vi "Open.vi"(7 "I2C Channel":u8, 8 "Error In":errorcluster, 10 "I2C Slave Address (0)":u8, 11 "LINX Resource":T1) -> (0 "Error Out":errorcluster, 2 "Success?":bool, 3 "LINX Resource":T1)   [LabVIEW 2020, in "LMH-LINX.lvlib" / "MMA8451.lvlib"]
doc: "Open the I2C master and initialize the MMA8451 accelerometer with 14-bit resolution and +-2g mode.\n\nIf the LINX device has more than one I2C master the logical first I2C master is channel 0, the next is channel 1, etc.\n\nOrignal code contributed by SEbstein."
uses:
  MMA8451.lvlib
  Private/Type Defs/LINX Ref.ctl
  Private/Type Defs/Platform.ctl
  Private/Type Defs/Interface.ctl
  Private/Device/Type Defs/LINX Device Config.ctl
  Private/Device/Type Defs/TCP Config.ctl
  Private/Device/Type Defs/Channels.ctl
  Private/Type Defs/Peripherals/I2C/EOF.ctl
  Private/Local IO/LinxI2cWrite.vi
  Utilities/Check Channel.vi
  Private/Utilties/Generate Error.vi
  LMH-LINX.lvlib
  Private/Device/Device.lvlib
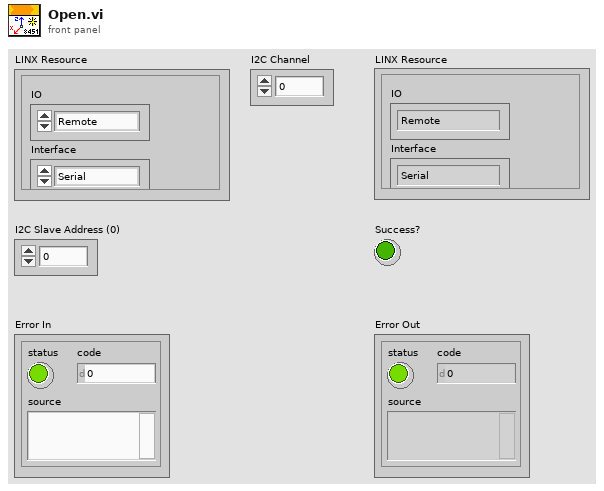
[diagram p1: front panel]
types:
  T1 = typedef "LMH-LINX.lvlib/LINX Ref.ctl" = cluster{"IO":T2, "Interface":T3, "LINX Device Config":T4}
  T2 = typedef "LMH-LINX.lvlib/Platform.ctl" = enum16{"Remote", "Local"}
  T3 = typedef "LMH-LINX.lvlib/Interface.ctl" = enum16{"Serial", "TCP"}
  T4 = typedef "Device.lvlib/LINX Device Config.ctl" = cluster{"Interface":T3, "COM Port":refnum<visa-resource-name>, "TCP Configuration":T5, "Device Family":u8, "Device ID":u8, "Device Name":string, "TCP Ref":refnum<k5>, "Channels":T6}
  T5 = typedef "Device.lvlib/TCP Config.ctl" = cluster{"IP Address":string, "Port":u16}
  T6 = typedef "LMH-LINX.lvlib/Channels.ctl" = cluster{"DI":u8[], "DO":u8[], "AI":u8[], "AO":u8[], "PWM":u8[], "QE":u8[], "UART":u8[], "I2C 2":u8[], "SPI":u8[], "CAN":u8[], "Servo":u8[], "AI Ref (V)":dbl, "AI Resolution (Bits)":u8, "AO Ref (V)":dbl, "AO Resolution (Bits)":u8}
  T7 = typedef "LMH-LINX.lvlib/EOF.ctl" = enum8{"Stop", "Restart", "Restart No Stop", "No Stop"}
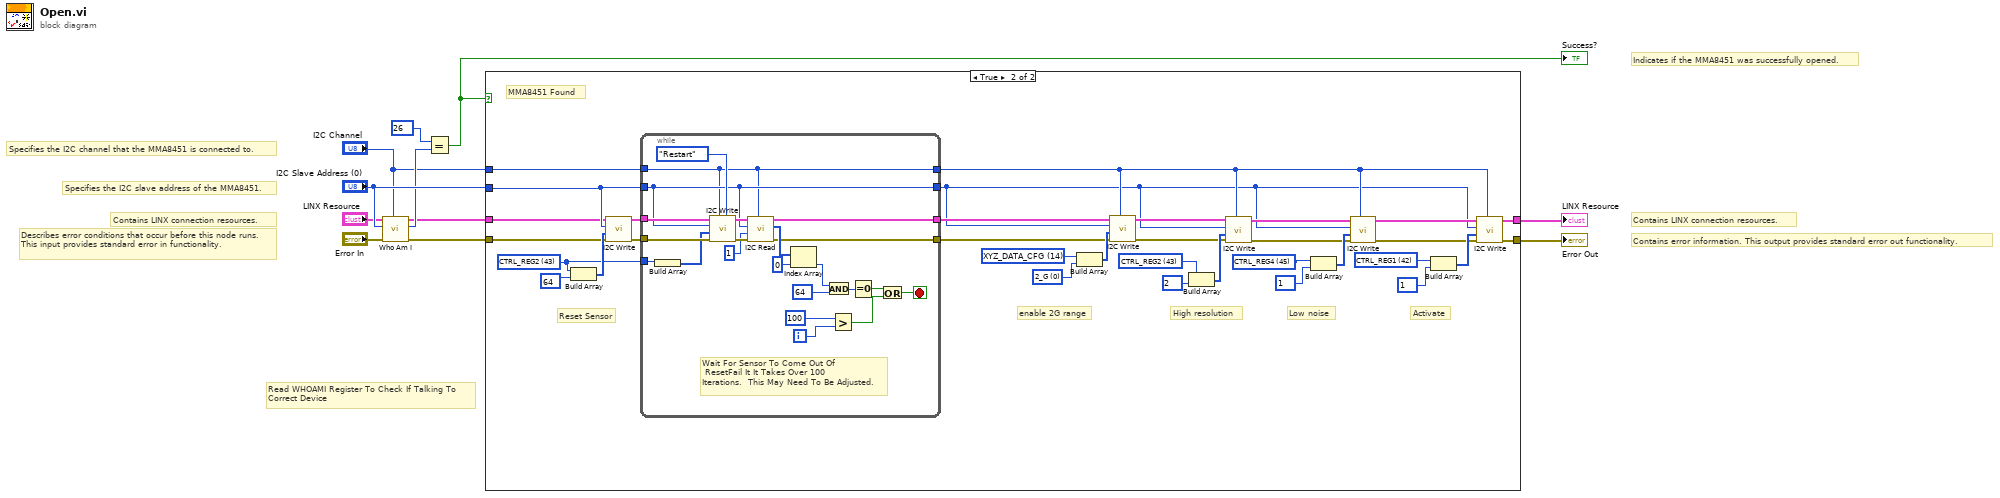
[diagram p0: block diagram]
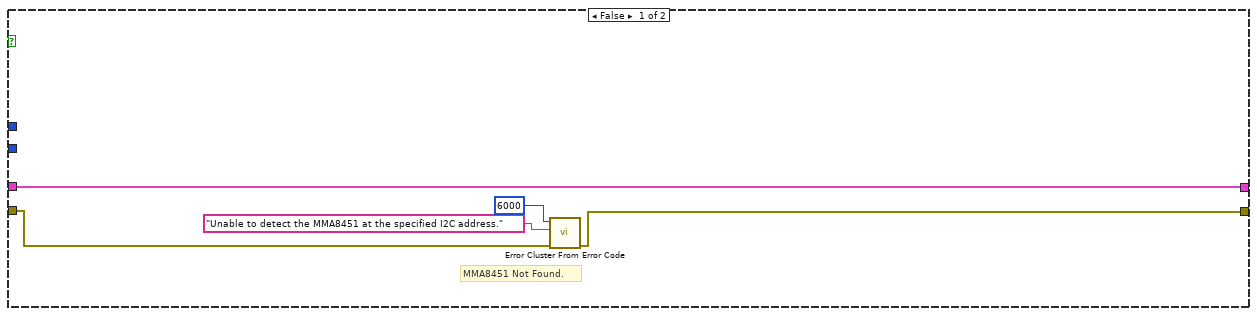
[diagram p2: hidden frame]
diagram:
  # "Indicates if the MMA8451 was successfully opened."
  # "Contains LINX connection resources."
  # "Contains error information. This output provides standard error out functionality."
  # "Specifies the I2C slave address of the MMA8451."
  # "Specifies the I2C channel that the MMA8451 is connected to."
  # "Contains LINX connection resources."
  # "Describes error conditions that occur before this node runs. This input provides standard error in functionality."
  # "Read WHOAMI Register To Check If Talking To \nCorrect Device"
  n1 = call "Who Am I.vi"("I2C Channel"="I2C Channel", "Error In"="Error In", "I2C Slave Address (0)"="I2C Slave Address (0)", "LINX Resource"="LINX Resource") -> ("Error Out"=w6:errorcluster, "ID"=w5:u8, "LINX Resource"=w3:T1)  [unwired: 5 in]
  n2 = Equal?(x=26, y=w5) -> (x = y?=w9:bool)
  "Success?" <- w9
  n3 = case shown="True" w9 {
    tunnel: [w14 w18] -> w10
    tunnel: "I2C Slave Address (0)" -> [_ w44]
    tunnel: w6 -> [w15 w47]
    tunnel: w3 -> [w16 w36]
    tunnel: "I2C Channel" -> [_ w35]
    tunnel: [w16 w17] -> w1
    frame False {
      # "MMA8451 Not Found."
      n4 = call <vilib>:"Error Cluster From Error Code.vi"("error in (no error)"=w15, "error message (\"\")"="Unable to detect the MMA8451 at the specified I2C address." ("error message (\"\")"), "error code (0)"=6000) -> ("error out"=w14:errorcluster)  [unwired: 6 in]
    }
    frame True {
      w25 = u8 42 items=["OUT_X_MSB"=1, "SYSMOD"=11, "WHOAMI"=13, "XYZ_DATA_CFG"=14, "PL_STATUS"=16, "PL_CFG"=17, "CTRL_REG1"=42, "CTRL_REG2"=43, "CTRL_REG4"=45, "CTRL_REG5"=46] ("MMA8451 REG_CTRL_REG1")
      w28 = u8 45 items=["OUT_X_MSB"=1, "SYSMOD"=11, "WHOAMI"=13, "XYZ_DATA_CFG"=14, "PL_STATUS"=16, "PL_CFG"=17, "CTRL_REG1"=42, "CTRL_REG2"=43, "CTRL_REG4"=45, "CTRL_REG5"=46] ("MMA8451 REG_CTRL_REG4")
      w33 = u8 43 items=["OUT_X_MSB"=1, "SYSMOD"=11, "WHOAMI"=13, "XYZ_DATA_CFG"=14, "PL_STATUS"=16, "PL_CFG"=17, "CTRL_REG1"=42, "CTRL_REG2"=43, "CTRL_REG4"=45, "CTRL_REG5"=46] ("MMA8451 REG_CTRL_REG2")
      w43 = u8 0 items=["8_G"=2, "4_G"=1, "2_G"=0] ("MMA8451 Range 2G")
      w42 = u8 14 items=["OUT_X_MSB"=1, "SYSMOD"=11, "WHOAMI"=13, "XYZ_DATA_CFG"=14, "PL_STATUS"=16, "PL_CFG"=17, "CTRL_REG1"=42, "CTRL_REG2"=43, "CTRL_REG4"=45, "CTRL_REG5"=46] ("MMA8451 XYZ_DATA_CFG")
      w34 = u8 43 items=["OUT_X_MSB"=1, "SYSMOD"=11, "WHOAMI"=13, "XYZ_DATA_CFG"=14, "PL_STATUS"=16, "PL_CFG"=17, "CTRL_REG1"=42, "CTRL_REG2"=43, "CTRL_REG4"=45, "CTRL_REG5"=46] ("MMA8451 REG_CTRL_REG2")
      # "Activate"
      # "Low noise"
      # "High resolution"
      # "enable 2G range"
      # "Reset Sensor"
      # "MMA8451 Found"
      n5 = Build Array(w34, u8 64 ("element")) -> (w48:u8[])
      n6 = call "I2C Write.vi"("Error In"=w47, "Data"=w48, "I2C Slave Address (0)"=w44, "LINX Resource"=w36) -> ("Error Out"=w45:errorcluster, "LINX Resource"=w46:T1)  [unwired: 6 in]
      n7 = while {
        tunnel: w46 -> [w64]
        tunnel: w45 -> [w65]
        tunnel: w44 -> [w51]
        tunnel: w35 -> [w50]
        tunnel: w34 -> [w63]
        tunnel: [w55] -> w31
        tunnel: [w54] -> w32
        tunnel: [w51] -> w19
        tunnel: [w50] -> w20
        i -> [w70]
        stop <- w66 stop-if-true
        # "Wait For Sensor To Come Out Of\n ResetFail It It Takes Over 100 \nIterations.  This May Need To Be Adjusted."
        n8 = Build Array(w63) -> (w62:u8[])
        n9 = call "I2C Write.vi"("EOF"=EOF."Restart", "I2C Channel"=w50, "Error In"=w65, "Data"=w62, "I2C Slave Address (0)"=w51, "LINX Resource"=w64) -> ("Error Out"=w59:errorcluster, "LINX Resource"=w60:T1)  [unwired: 4 in]
        n10 = call "I2C Read.vi"("I2C Channel"=w50, "Error In"=w59, "Bytes To Read"=u8 1, "I2C Slave Address (0)"=w51, "LINX Resource"=w60) -> ("Error Out"=w55:errorcluster, "Data"=w56:u8[], "LINX Resource"=w54:T1)  [unwired: 4 in]
        n11 = Index Array(array=w56, index=0) -> (element=w53:u8)
        n12 = And(x=w53, y=u8 64) -> (x .and. y?=w71:u8)
        n13 = Greater?(x=100, y=w70) -> (0:w68:bool)
        n14 = Equal To 0?(x=w71) -> (x = 0?=w67:bool)
        n15 = Or(x=w67, y=w68) -> (x .or. y?=w66:bool)
      }
      n16 = Build Array(w42, w43) -> (w41:u8[])
      n17 = call "I2C Write.vi"("I2C Channel"=w20, "Error In"=w31, "Data"=w41, "I2C Slave Address (0)"=w19, "LINX Resource"=w32) -> ("Error Out"=w37:errorcluster, "LINX Resource"=w38:T1)  [unwired: 5 in]
      n18 = Build Array(w33, u8 2 ("element")) -> (w39:u8[])
      n19 = call "I2C Write.vi"("I2C Channel"=w20, "Error In"=w37, "Data"=w39, "I2C Slave Address (0)"=w19, "LINX Resource"=w38) -> ("Error Out"=w27:errorcluster, "LINX Resource"=w26:T1)  [unwired: 5 in]
      n20 = Build Array(w28, u8 1 ("element")) -> (w30:u8[])
      n21 = call "I2C Write.vi"("I2C Channel"=w20, "Error In"=w27, "Data"=w30, "I2C Slave Address (0)"=w19, "LINX Resource"=w26) -> ("Error Out"=w22:errorcluster, "LINX Resource"=w21:T1)  [unwired: 5 in]
      n22 = Build Array(w25, u8 1 ("element")) -> (w23:u8[])
      n23 = call "I2C Write.vi"("I2C Channel"=w20, "Error In"=w22, "Data"=w23, "I2C Slave Address (0)"=w19, "LINX Resource"=w21) -> ("Error Out"=w18:errorcluster, "LINX Resource"=w17:T1)  [unwired: 5 in]
    }
  }
  "Error Out" <- w10
  "LINX Resource" <- w1
